vi "8.3 Single-channel Acquisition Data Types.vi"() -> ()   [LabVIEW 2019]
uses:
  <vilib>/DAQmx/read.llb/DAQmx Read (Analog Wfm 1Chan NSamp).vi
  <vilib>/DAQmx/create/channels.llb/DAQmx Create Channel (AI-Voltage-Basic).vi
  <vilib>/DAQmx/configure/timing.llb/DAQmx Timing (Sample Clock).vi
  <vilib>/DAQmx/miscellaneous.llb/DAQmx Fill In Error Info.vi
  <resource>/objmgr/daqmx.rc
panel:
  out "wavform indicator":waveform(dbl)
  out "Graph":waveform(dbl)(graph)
  out "Chart":waveform(dbl)(graph)
  in  "Stop":bool
  out "Actual Sample Rate (Hz)":dbl
  in  "Configuration Control":T1={"number of samples"=-1, "Minimum Value"=-1.0, "Maximum Value"=-1.0, "physical channels"="Multi_I-O/ai0", "Desired Sample Rate (Hz)"=-1.0, "sample mode"=10178} {"sample mode" items=["Finite Samples"=10178, "Continuous Samples"=10123, "Hardware Timed Single Point"=12522]}
  # "Full DAQmx API"
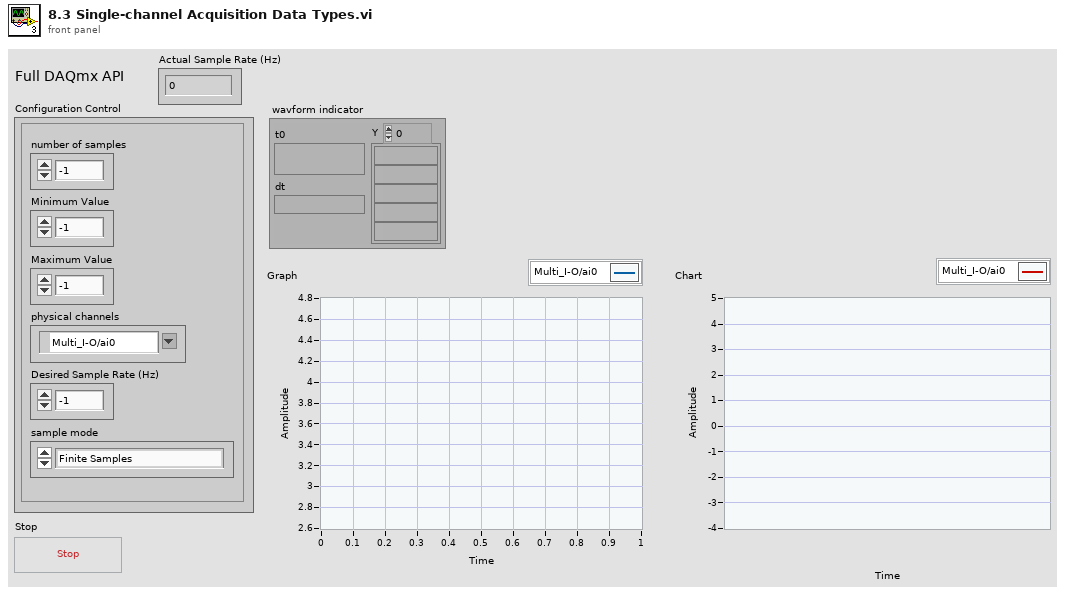
[diagram p1: front panel]
types:
  T1 = cluster{"number of samples":i32, "Minimum Value":dbl, "Maximum Value":dbl, "physical channels":tag, "Desired Sample Rate (Hz)":dbl, "sample mode":i32}
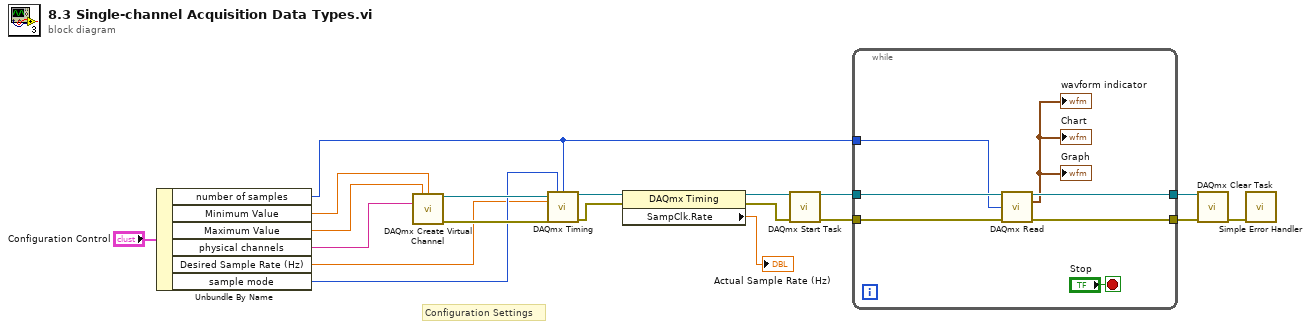
[diagram p0: block diagram]
diagram:
  # "Configuration Settings"
  n1 = Unbundle By Name("Configuration Control") -> ("number of samples"=w4:i32, "Minimum Value"=w15:dbl, "Maximum Value"=w16:dbl, "physical channels"=w14:tag, "Desired Sample Rate (Hz)"=w12:dbl, "sample mode"=w13:i32)
  n2 = call-poly <vilib>:"DAQmx Create Virtual Channel.vi"("maximum value"=w16, "minimum value"=w15, "physical channels"=w14) -> ("task out"=w19:refnum<k21>, "error out"=w18:errorcluster)  [unwired: 11 in]
  n3 = call-poly <vilib>:"DAQmx Timing.vi"("task/channels in"=w19, "sample mode"=w13, "samples per channel"=w4, "rate"=w12, "error in"=w18) -> ("task out"=w10:refnum<k21>, "error out"=w11:errorcluster)  [unwired: 9 in]
  n4 = property class="DAQmx Timing"(reference=w10, error in=w11) -> (reference out=w7:refnum<k21>, error out=w6:errorcluster, "SampClk.Rate"=→"Actual Sample Rate (Hz)":dbl)
  n5 = call <vilib>:"DAQmx Start Task.vi"("task/channels in"=w7, "error in"=w6) -> ("task out"=w8:refnum<k21>, "error out"=w5:errorcluster)  [unwired: 12 in]
  n6 = while {
    tunnel: w8 -> [w26]
    tunnel: w5 -> [w25]
    tunnel: w4 -> [w24]
    tunnel: [w22] -> w2
    tunnel: [w21] -> w1
    stop <- "Stop" stop-if-true
    n7 = call-poly <vilib>:"DAQmx Read.vi"("task/channels in"=w26, "number of samples per channel"=w24, "error in"=w25) -> ("task out"=w22:refnum<k21>, "data"=→"Chart" →"Graph" →"wavform indicator":waveform(dbl), "error out"=w21:errorcluster)  [unwired: 10 in]
  }
  n8 = call <vilib>:"DAQmx Clear Task.vi"("task in"=w2, "error in"=w1) -> ("error out"=w3:errorcluster)  [unwired: 13 in]
  n9 = call <vilib>:"Simple Error Handler.vi"("error in (no error)"=w3) -> ()  [unwired: 4 in, 5 out]
